vi "visual.vi"(2 "Attributes":T1) -> (4 "urdf out":string)   [LabVIEW 2010]
uses:
  VisionAttributes.ctl
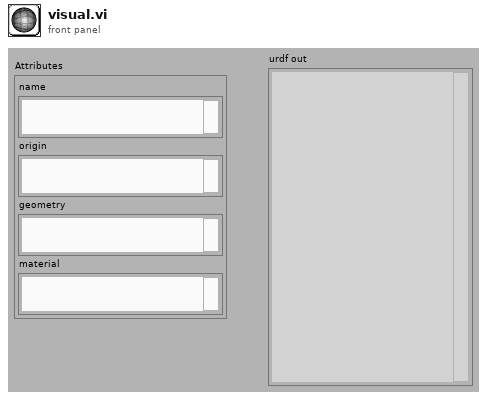
[diagram p1: front panel]
types:
  T1 = typedef "VisionAttributes.ctl" = cluster{"name":string, "origin":string, "geometry":string, "material":string}
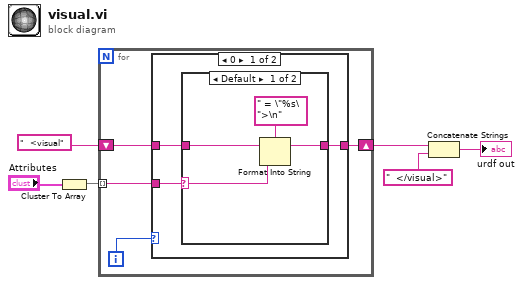
[diagram p0: block diagram]
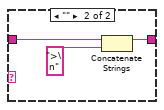
[diagram p2: hidden frame]
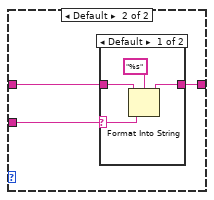
[diagram p3: hidden frame]
diagram:
  n1 = Cluster To Array(cluster="Attributes") -> (array=w6:string[])
  n2 = for {
    shift-right: [w10] -> w5
    shift-left: "  <visual" -> [w9]
    tunnel: w6 -> [w8] mode=indexing
    i -> [w7]
    n3 = case shown="0" w7 {
      tunnel: [w11 w23] -> w10
      tunnel: w9 -> [w12 w22]
      tunnel: w8 -> [w13 w21]
      frame 0 {
        n4 = case shown="Default" w13 {
          selector: w13 -> [w14 _]
          tunnel: w12 -> [w16 w19]
          tunnel: [w15 w18] -> w11
          frame Default {
            n5 = Format Into String(format string=" = \"%s\">\n", initial string=w16, w14) -> (resulting string=w15:string)  [unwired: 1 in, 1 out]
          }
          frame "" {
            n6 = Concatenate Strings(w19, ">\n") -> (w18:string)
          }
        }
      }
      frame Default {
        n7 = case shown="Default" w21 {
          selector: w21 -> [w25 _]
          tunnel: [w24 w28] -> w23
          tunnel: w22 -> [w27 w28]
          frame Default {
            n8 = Format Into String(format string="%s", initial string=w27, w25) -> (resulting string=w24:string)  [unwired: 1 in, 1 out]
          }
          frame "" {
          }
        }
      }
    }
  }
  n9 = Concatenate Strings(w5, "  </visual>") -> (→"urdf out":string)
